vi "Solve Center Wavelength.vi"(4 "Standard Wavelength":dbl=500.0 format="%#_8g", 6 "Current Central Wavelength":dbl=600.0 format="%#_8g", 7 "pixel index":dbl=200.0 min=0.0 max=1024.0 format="%.2f", 8 "File Info":T1={"FilePath"=path "/Opticsmac/Documents/Data", "Field (T)"=55.0, "Temperature (K)"=77.0, "X-Axis"=enum."nm", "Center nm"=600.0, "Current Grating Density"=enum."600", "CCD Parameters"={"Exposure Time (s)"=0.2, "Offset"=0.0, "BkgrdCrct"=FALSE, "Shutter"=FALSE, "Mode"=enum."Regular", "Repetition"=4, "dt or s"=0.0}, "Operation Mode"=enum."NML Data Acquisition", "Exp Index"=0, "Index_repetition"=0, "Index"=0, "Current Detector"=enum."CCD-1024x256"} {"CCD Parameters"."dt or s" format="%#.6f"; "CCD Parameters"."Repetition" min=1; "CCD Parameters"."Offset" format="%#.2f"; "CCD Parameters"."Exposure Time (s)" min=0.02 max=6000.0 format="%#.2f"; "Center nm" format="%.2f"; "Temperature (K)" format="%.2f"; "Field (T)" format="%.2f"}) -> (3 "Solved Central Wavelength for Calibration":dbl=517.6607981427933 format="%.4f")   [LabVIEW 2024]
uses:
  Globals and TypeDefs/Type Definitions.llb/FileInfoParameter.ctt
  Globals and TypeDefs/Type Definitions.llb/Wavelength Unit.ctt
  Globals and TypeDefs/Type Definitions.llb/McPherson Grating Density.ctl
  Globals and TypeDefs/Type Definitions.llb/CCDParameter.ctt
  Globals and TypeDefs/Type Definitions.llb/OperationMode.ctt
  Globals and TypeDefs/Type Definitions.llb/ListOfDetectors.ctt
panel:
  out "Last iteration delta":dbl=2.3305801732931286e-12 format="%.2e"
  out "Iterations needed":i32=4
  in  "Maximum Iterations":u16=1000
  out "1st iteration Wavelength":dbl=582.5031806844609 format="%.4f"
  in  "Tolerance":dbl=1e-10 format="%.2e"
  out "Self-Consistent Standard Wavelength":dbl=499.99999999999767 format="%.4f"
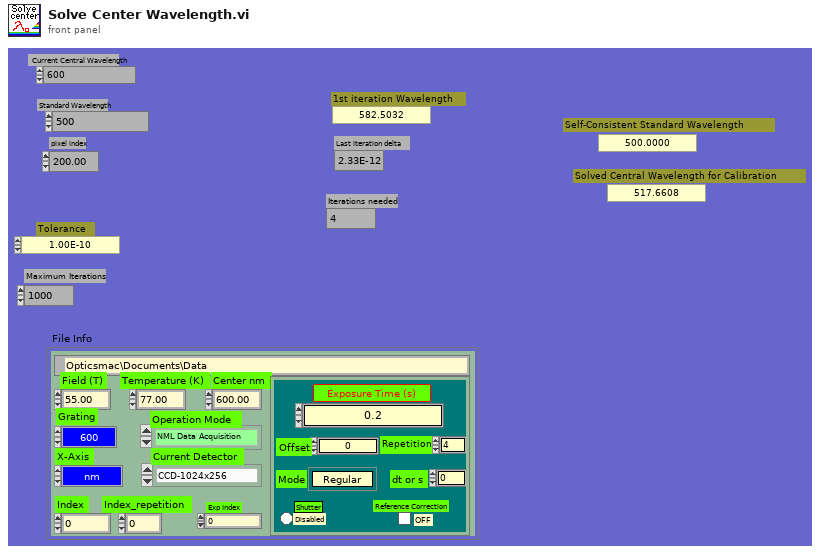
[diagram p1: front panel]
types:
  T1 = typedef "FileInfoParameter.ctt" = cluster{"FilePath":path, "Field (T)":dbl, "Temperature (K)":dbl, "X-Axis":T2, "Center nm":dbl, "Current Grating Density":T3, "CCD Parameters":T4, "Operation Mode":T5, "Exp Index":u32, "Index_repetition":u16, "Index":u16, "Current Detector":T6}
  T2 = typedef "Wavelength Unit.ctt" = enum8{"Point", "nm", "eV", "meV", "cm_1"}
  T3 = typedef "McPherson Grating Density.ctl" = enum8{"150", "300", "600", "1200", "1800"}
  T4 = typedef "CCDParameter.ctt" = cluster{"Exposure Time (s)":dbl, "Offset":dbl, "BkgrdCrct":bool, "Shutter":bool, "Mode":enum8{"Regular", "OverExp Cor", "SpikeRemove", "ForCalibration"}, "Repetition":u16, "dt or s":dbl}
  T5 = typedef "OperationMode.ctt" = enum16{"Standby", "CCD Single Shot", "CCD Sequence Shots", "CCD Custom Shots", "CCD Reference Shot", "Step Scanning ", "Time Scanning", "NML Data Acquisition"}
  T6 = typedef "ListOfDetectors.ctt" = enum8{"CCD-1024x256", "InGaAs PDA-1024x1", "CCD-1340x400", "Ge Single Channel", "Si Single Channel", "PMT Single Channel"}
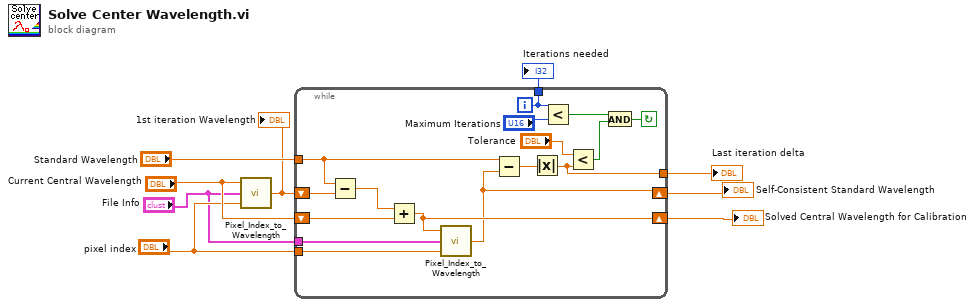
[diagram p0: block diagram]
diagram:
  n1 = call "Pixel_Index_to_Wavelength.vi"("pixel index"="pixel index", "File Info In"="File Info", "Central Wavelength"="Current Central Wavelength") -> ("nm (out)"=w3:dbl)  [unwired: 2 in]
  "1st iteration Wavelength" <- w3
  n2 = while {
    tunnel: [w10] -> w1
    tunnel: [w11] -> w2
    tunnel: "Standard Wavelength" -> [w19]
    shift-left: "Current Central Wavelength" -> [w24]
    shift-right: [w21] -> w7
    tunnel: "pixel index" -> [w22]
    tunnel: "File Info" -> [w23]
    shift-left: w3 -> [w25]
    shift-right: [w18] -> w8
    i -> [w11]
    stop <- w14 continue-if-true
    n3 = Subtract(x=w19, y=w25) -> (x-y=w20:dbl)
    n4 = Add(x=w20, y=w24) -> (x+y=w21:dbl)
    n5 = call "Pixel_Index_to_Wavelength.vi"("pixel index"=w22, "File Info In"=w23, "Central Wavelength"=w21) -> ("nm (out)"=w18:dbl)  [unwired: 2 in]
    n6 = Subtract(x=w19, y=w18) -> (x-y=w17:dbl)
    n7 = Absolute Value(x=w17) -> (abs(x)=w10:dbl)
    n8 = Less?(x=w11, y="Maximum Iterations") -> (x < y?=w13:bool)
    n9 = Less?(x="Tolerance", y=w10) -> (x < y?=w12:bool)
    n10 = And(x=w13, y=w12) -> (x .and. y?=w14:bool)
  }
  "Solved Central Wavelength for Calibration" <- w7
  "Self-Consistent Standard Wavelength" <- w8
  "Iterations needed" <- w2
  "Last iteration delta" <- w1
